vi "get_objectArray.vi"(0 "HGF_ThreadTask":refnum<class "HGF_ThreadTask.lvclass">, 5 "error in (no error)":errorcluster) -> (14 "dup HGF_ThreadTask":refnum<class "HGF_ThreadTask.lvclass">, 16 "objectArray":refnum<class>[](array[class]), 17 "errorArray":errorcluster[](array[cluster]), 19 "error out":errorcluster)   [LabVIEW 2014, in "HGF_BaseClasses.lvlib" / "HGF_ThreadTask.lvclass"]
doc: "Read object array."
uses:
  HGF_ThreadTask.lvclass
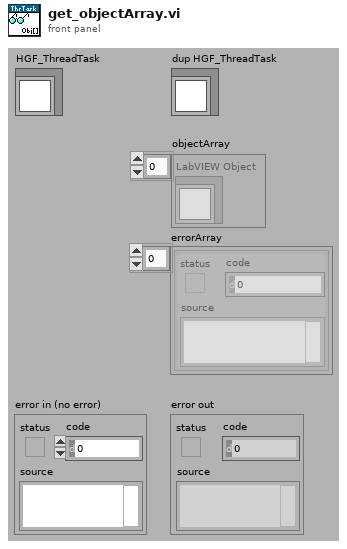
[diagram p1: front panel]
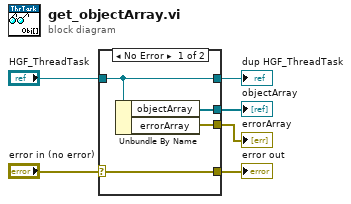
[diagram p0: block diagram]
diagram:
  n1 = case shown="No Error" "error in (no error)" {
    selector: "error in (no error)" -> [w10 w11]
    tunnel: [w10 w11] -> w5
    tunnel: [w9 w12] -> w3
    tunnel: "HGF_ThreadTask" -> [w9 w12]
    tunnel: [w8 _] -> w2
    tunnel: [w7 _] -> w1
    frame No Error {
      n2 = Unbundle By Name(w9) -> ("objectArray"=w8:refnum<class>[], "errorArray"=w7:errorcluster[])
    }
    frame Error {
    }
  }
  "error out" <- w5
  "dup HGF_ThreadTask" <- w3
  "objectArray" <- w2
  "errorArray" <- w1
